vi "Set speed.vi"(8 "error in (no error)":errorcluster, 11 "StageSPIM in":refnum<class "StageSPIM.lvclass">) -> (0 "error out":errorcluster, 3 "StageSPIM out":refnum<class "StageSPIM.lvclass">)   [LabVIEW 2012, in "StageSPIM.lvclass"]
uses:
  StageSPIM.lvclass
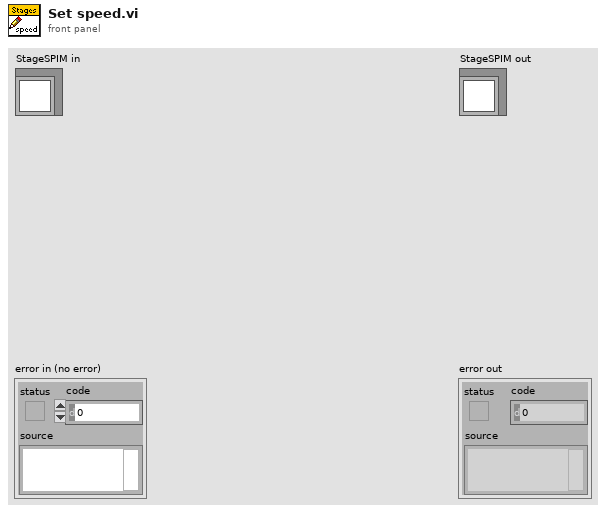
[diagram p1: front panel]
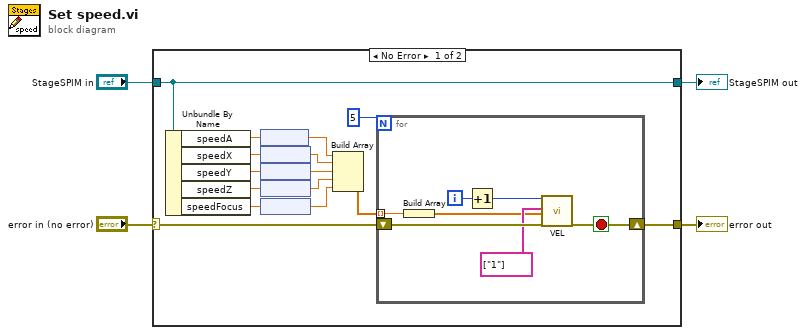
[diagram p0: block diagram]
diagram:
  n1 = case shown="No Error" "error in (no error)" {
    selector: "error in (no error)" -> [w19 w28]
    tunnel: [w18 w28] -> w3
    tunnel: [w16 w27] -> w1
    tunnel: "StageSPIM in" -> [w16 w27]
    frame No Error {
      n2 = Unbundle By Name(w16) -> ("speedA"=w13:dbl[unit], "speedX"=w12:dbl[unit], "speedY"=w15:dbl[unit], "speedZ"=w14:dbl[unit], "speedFocus"=w7:dbl[unit])
      n3 = node(w13) -> (w11:dbl)
      n4 = node(w12) -> (w6:dbl)
      n5 = node(w15) -> (w10:dbl)
      n6 = node(w14) -> (w9:dbl)
      n7 = node(w7) -> (w5:dbl)
      n8 = Build Array(w11, w6, w10, w9, w5) -> (w8:dbl[])
      n9 = for {
        N: 5 -> [_]
        shift-right: [w22] -> w18
        shift-left: w19 -> [w26]
        tunnel: w8 -> [w21] mode=indexing
        i -> [w24]
        stop <- w22 stop-if-true
        n10 = Build Array(w21) -> (w20:dbl[])
        n11 = Increment(x=w24) -> (x+1=w23:i32)
        n12 = call "VEL.vi"("System no."=w23, "Axes to set"=string[] ["1"], "Velocity values"=w20, "error in"=w26) -> ("error out"=w22:errorcluster)  [unwired: 14 in, 1 out]
      }
    }
    frame Error {
    }
  }
  "error out" <- w3
  "StageSPIM out" <- w1
